vi "build.vi"(8 "error in (no error)":errorcluster, 10 "build_spec":T1, 11 "lv-builder-l3 in":refnum<class "lv-builder-l3.lvclass">) -> (0 "error out":errorcluster, 2 "[] generated_files":path[](array[path]), 3 "lv-builder-l3 out":refnum<class "lv-builder-l3.lvclass">)   [LabVIEW 2015, in "lv-builder-l3.lvlib" / "lv-builder-l3.lvclass"]
uses:
  lv-builder-l3.lvclass
  lv-build/public/_controls/build_specification.ctl
  lv-build/public/_controls/build_type.ctl
  <vilib>/AppBuilder/AB_API_Simple/Build (path).vi
  <vilib>/AppBuilder/AB_API_Simple/NI_App_Builder_API.lvlib
  lv-build/lv-build.lvlib
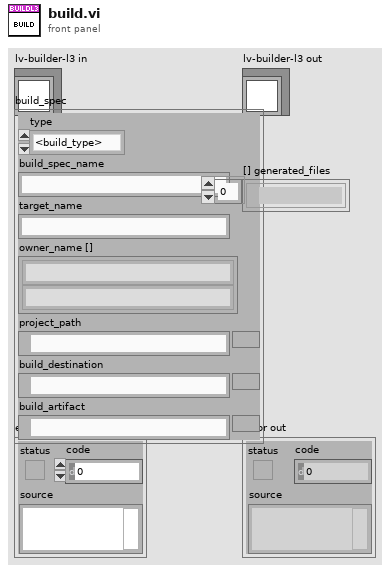
[diagram p1: front panel]
types:
  T1 = typedef "lv-build.lvlib/build_specification.ctl" = cluster{"type":T2, "build_spec_name":string, "target_name":string, "owner_name []":string[], "project_path":path, "build_destination":path, "build_artifact":path}
  T2 = typedef "lv-build.lvlib/build_type.ctl" = enum16{"<build_type>", "application_pc", "application_rt", "installer", "llb", "lvlibp", "zip", "fpga", "<null>"}
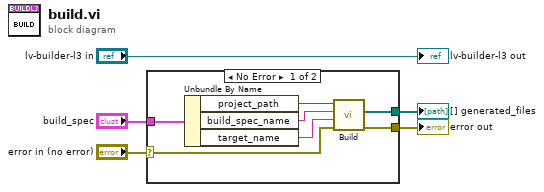
[diagram p0: block diagram]
diagram:
  n1 = case shown="No Error" "error in (no error)" {
    selector: "error in (no error)" -> [w8 w13]
    tunnel: "build_spec" -> [w12 _]
    tunnel: [w7 w13] -> w3
    tunnel: [w6 _] -> w1
    frame No Error {
      n2 = Unbundle By Name(w12) -> ("project_path"=w11:path, "build_spec_name"=w10:string, "target_name"=w9:string)
      n3 = call-poly <vilib>:"Build.vi"("error in (no error)"=w8, "Name of target (My Computer)"=w9, "Name of build specification (if empty: build all)"=w10, "Path to project"=w11) -> ("error out"=w7:errorcluster, "Generated files"=w6:path[])  [unwired: 6 in]
    }
    frame Error {
    }
  }
  "error out" <- w3
  "[] generated_files" <- w1
  "lv-builder-l3 out" <- "lv-builder-l3 in"
